vi "playSound.vi"(8 "error in (no error)":errorcluster, 11 "Sound in":refnum<class "Sound.lvclass">) -> (0 "error out":errorcluster, 3 "Sound out":refnum<class "Sound.lvclass">)   [LabVIEW 2020, in "Sound.lvclass"]
uses:
  Sound.lvclass
  Sound.lvclass/Sound.ctl
  <vilib>/sound2/lvsound2.llb/Sound Output Write (DBL Single).vi
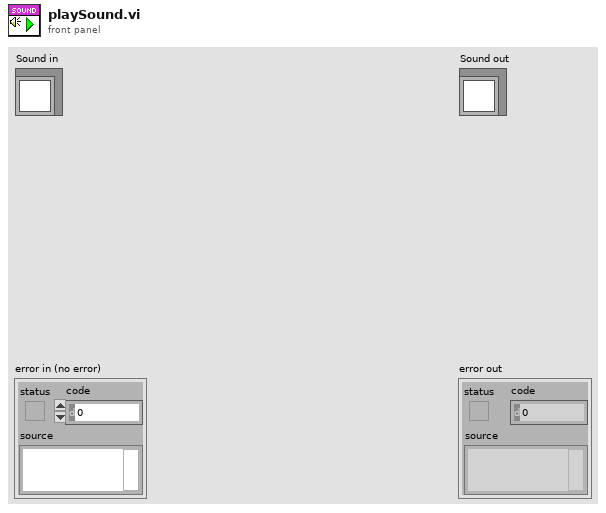
[diagram p1: front panel]
types:
  T1 = typedef "Sound Output Task ID.ctl" = u32
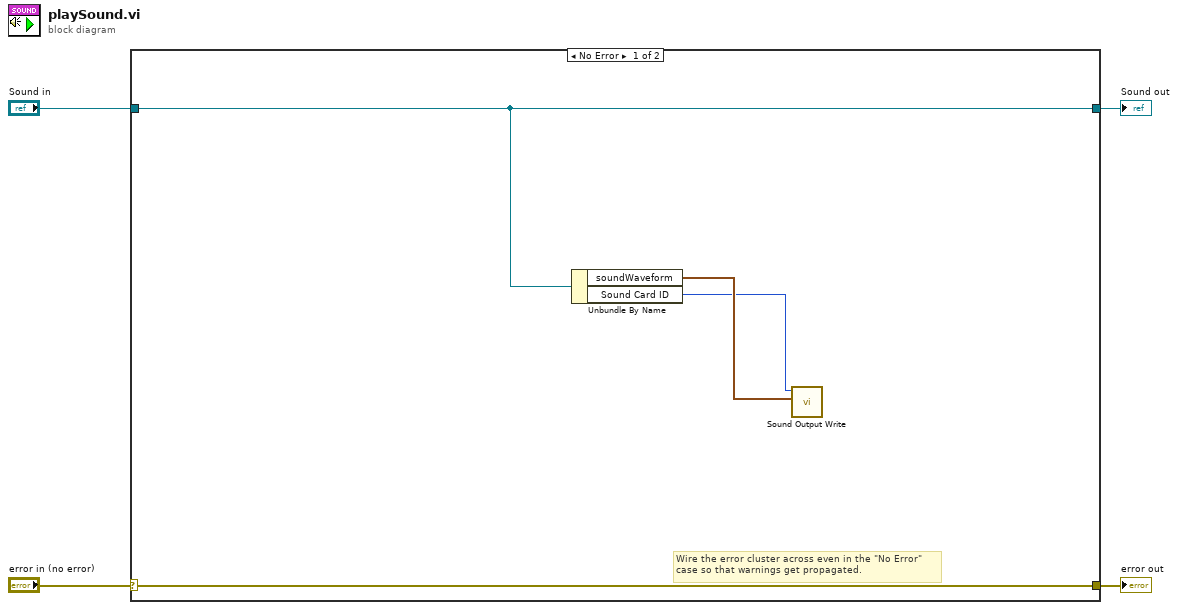
[diagram p0: block diagram]
diagram:
  n1 = case shown="No Error" "error in (no error)" {
    selector: "error in (no error)" -> [w8 w10]
    tunnel: [w8 w10] -> w3
    tunnel: [w7 w9] -> w1
    tunnel: "Sound in" -> [w7 w9]
    frame No Error {
      # "Wire the error cluster across even in the \"No Error\"\ncase so that warnings get propagated."
      n2 = Unbundle By Name(w7) -> ("soundWaveform"=w6:waveform(dbl), "Sound Card ID"=w5:T1)
      n3 = call-poly <vilib>:"Sound Output Write.vi"("data"=w6, "task ID"=w5) -> ()  [unwired: 8 in, 2 out]
    }
    frame Error {
    }
  }
  "error out" <- w3
  "Sound out" <- w1
